vi "Speaker DMA Transfer.vi"   [LabVIEW 2018]
doc: "Handle changes to the speaker signal here. The speaker signal is stored in the memory labeled <b>Speaker Signal</b>. The host may change the speaker signal by writing to the DMA FIFO <b>Speaker Data DMA</b>. The memory expects 40k elements."
uses:
  <vilib>/rvi/Emulation/niFpgaGetClockAttributes.vi
  <vilib>/rvi/Emulation/niFpgaSctlEmulationGetInTimedLoop.vi
  <vilib>/rvi/Emulation/niFpgaEmulationReportErrorSimple.vi
  <vilib>/rvi/Emulation/niFpgaEmulationIsFPGAContextNoSignature.vi
  <vilib>/rvi/DataTransferAndStorage/Container/Common/niFpgaContainerGetUniqueNameForEmu.vi
  <vilib>/rvi/Memory/Memory_Emulation/niFpgaMemoryEmulationCacheClearOnFirstRun.vi
  <vilib>/rvi/Memory/Memory_Emulation/nirvimemoryEmulationManagerCache_MakeExclusive.vi
  <vilib>/rvi/Memory/Memory_Emulation/niFpgaMemoryEmulationValidateCache.vi
  <vilib>/rvi/Memory/Memory_Emulation/nirvimemoryEmulationManagerCache_InsertValue.vi
  <vilib>/Utility/error.llb/Clear Errors.vi
  <vilib>/rvi/Memory/Memory_Emulation/nirvimemoryEmulationManagerCache_ReleaseExclusive.vi
  <vilib>/rvi/Memory/Memory_Emulation/nirvimemoryEmulationManagerCache_GetValue.vi
  <vilib>/rvi/Memory/Memory_Emulation/nirvimemoryEmulationManagerCache_SetValue.vi
  <vilib>/rvi/Emulation/niFpgaProcessEmulError.vi
  <vilib>/rvi/interface/RandomDataEmulation/niFpgaRandomDataHandleErrors.vi
  <vilib>/rvi/Memory/Memory_Emulation/nirvimemoryFastEmulation.vi
  <vilib>/rvi/Memory/Memory_Emulation/nirvimemoryEmulation.vi
  <vilib>/rvi/errors/nirviReportUnexpectedCaseInternalError (U32).vi
  <vilib>/rvi/Emulation/niFpgaCriticalErrorInLSC.vi
  <vilib>/rvi/DataTransferAndStorage/Container/XNode/niFpgaContainer.xnode
  <vilib>/rvi/DataTransferAndStorage/Register/Emulation/niFpgaRegisterEmulation.vi
  <vilib>/rvi/interface/RandomDataEmulation/nirviRandomDataFpgaReadWriteTemplate.vi
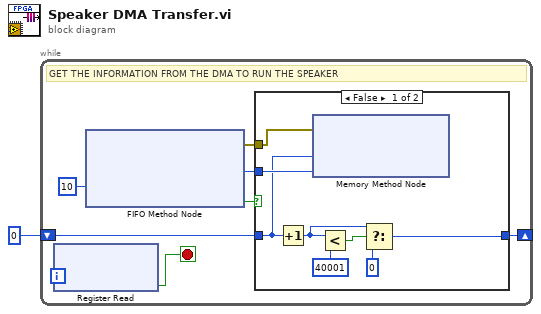
[diagram p0: block diagram]
diagram:
  n1 = while {
    shift-right: [w4] -> _
    shift-left: u32 0 ("Address") -> [w5]
    stop <- w2 stop-if-true
    # "GET THE INFORMATION FROM THE DMA TO RUN THE SPEAKER"
    n2 = xnode ("Register Read")() -> ("Data"=w2:bool)  [unwired: 1 in, 1 out]
    n3 = xnode ("FIFO Method Node")("Timeout"=10) -> ("Element"=w7:i16, "Timed Out?"=w6:bool, "error out"=w3:errorcluster)  [unwired: 2 in, 1 out]
    n4 = case shown="False" w6 {
      tunnel: w7 -> [w16 _]
      tunnel: w5 -> [w15 w17]
      tunnel: [w10 w17] -> w4
      tunnel: w3 -> [w9 _]
      frame False {
        n5 = Increment(x=w15) -> (x+1=w12:u32)
        n6 = xnode ("Memory Method Node")("Address"=w15, "Data"=w16, "error in (no error)"=w9) -> ()  [unwired: 1 in, 2 out]
        n7 = Less?(x=w12, y=u32 40001) -> (x < y?=w13:bool)
        n8 = Select(t=w12, s=w13, f=u32 0) -> (s? t:f=w10:u32)
      }
      frame True {
      }
    }
  }
